vi "Check if running.vi"(8 "error in (no error)":errorcluster, 11 "VI in":refnum<vi>) -> (0 "error out":errorcluster, 2 "Running?":bool, 3 "VI out":refnum<vi>)   [LabVIEW 2020, in "View Test.lvclass"]
uses:
  View Test.lvclass
  View Test.lvclass/View Test.ctl
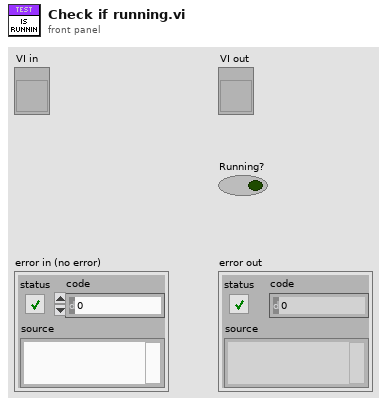
[diagram p1: front panel]
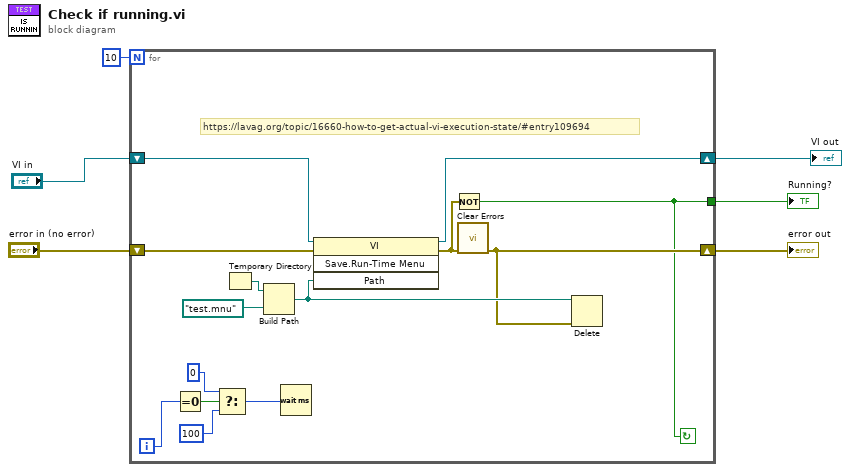
[diagram p0: block diagram]
diagram:
  n1 = for {
    N: 10 -> [_]
    tunnel: [w12] -> w6
    shift-right: [w13] -> w2
    shift-left: "error in (no error)" -> [w15]
    shift-right: [w20] -> w5
    shift-left: "VI in" -> [w14]
    i -> [w11]
    stop <- w12 continue-if-true
    # "https://lavag.org/topic/16660-how-to-get-actual-vi-execution-state/#entry109694"
    n2 = Equal To 0?(x=w11) -> (x = 0?=w8:bool)
    n3 = Select(t=u32 0 ("milliseconds to wait"), s=w8, f=u32 100 ("milliseconds to wait")) -> (s? t:f=w7:u32)
    n4 = Temporary Directory() -> (w16:path)
    n5 = Build Path(base path=w16, name or relative path=path "test.mnu") -> (appended path=w18:path)
    n6 = Wait (ms)(milliseconds to wait=w7) -> ()  [unwired: 1 out]
    n7 = invoke class="VI" method="Save.Run-Time Menu"(reference=w14, error in=w15, "Path"=w18) -> (reference out=w20:refnum<vi>, error out=w19:errorcluster)  [unwired: 1 in, 2 out]
    n8 = Not(x=w19) -> (.not. x?=w12:bool)
    n9 = call <vilib>:"Clear Errors.vi"("error in (no error)"=w19) -> ("error out"=w13:errorcluster)  [unwired: 5 in, 1 out]
    n10 = Delete(path (use dialog)=w18, error in=w13) -> ()  [unwired: 3 in, 3 out]
  }
  "error out" <- w2
  "Running?" <- w6
  "VI out" <- w5
